vi "Test Longer missmatch.vi"(11 "Test Case In":refnum<class "Find Index to Insert at Test.lvclass">) -> (0 "error out":errorcluster, 3 "Test Case Out":refnum<class "Find Index to Insert at Test.lvclass">)   [LabVIEW 2020, in "Find Index to Insert at Test.lvclass"]
uses:
  Find Index to Insert at Test.lvclass
  usr/local/natinst/LabVIEW-2026-64/vi.lib/Astemes/LUnit/Test Case.lvclass
  <vilib>/Astemes/LUnit/Test Case.lvclass/Test Case.ctl
  4993e8ee-a06a-463a-9684-69129f64d5ce.vi
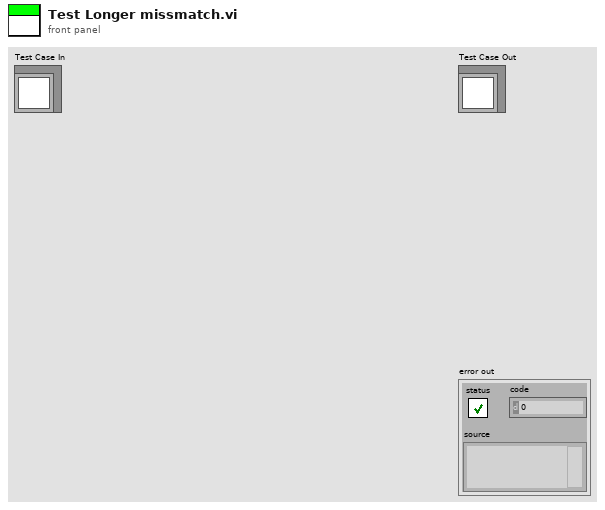
[diagram p1: front panel]
types:
  T1 = cluster{"Selection Start":u32, "Selection End":u32}[]
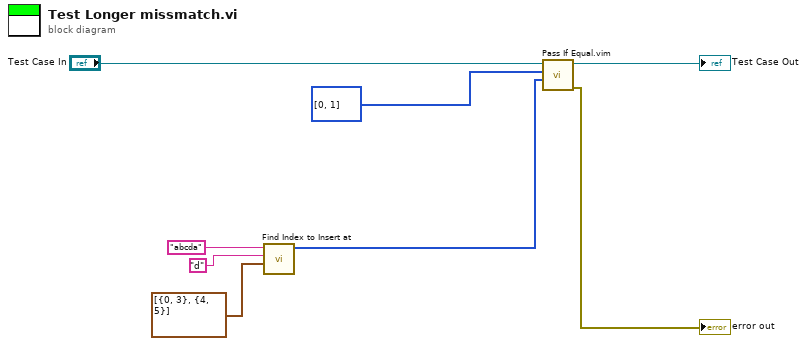
[diagram p0: block diagram]
diagram:
  n1 = call "Find Index to Insert at.vi"("Sections in Target"=T1 [{"Selection Start"=0, "Selection End"=3}, {"Selection Start"=4, "Selection End"=5}], "Reference"="d", "Target"="abcda") -> ("Indices in Ref"=w2:i32[])  [unwired: 8 in]
  n2 = call "Pass If Equal.vim"("Actual"=w2, "Expected"=i32[] [0, 1] ("Indices in Ref"), "LUnit Test Case In"="Test Case In") -> ("error out"=→"error out":errorcluster, "LUnit Test Case Out"=→"Test Case Out":refnum<class "Find Index to Insert at Test.lvclass">)  [unwired: 7 in]
